vi "sub_test_lut.vi"(9 "Calibration data":T1, 10 "Normalized axis positions":sgl[](array[numeric]) format="%#.4f", 11 "Error stop":sgl=50.0) -> (2 "Plausible point":bool, 3 "Error squared":sgl[](array[numeric]) format="%#.0f")   [LabVIEW 2012]
uses:
  initialization/asap_calibration.ctl
  <vilib>/Analysis/Matrix/Datatypes/RealMatrix.ctl
  <vilib>/Analysis/Matrix/NI_Matrix.lvlib
panel:
  out "Output f(x)":sgl[](array[numeric]) format="%#.0f"
  out "XYZ and match error":sgl[](array[numeric]) format="%#.0f"
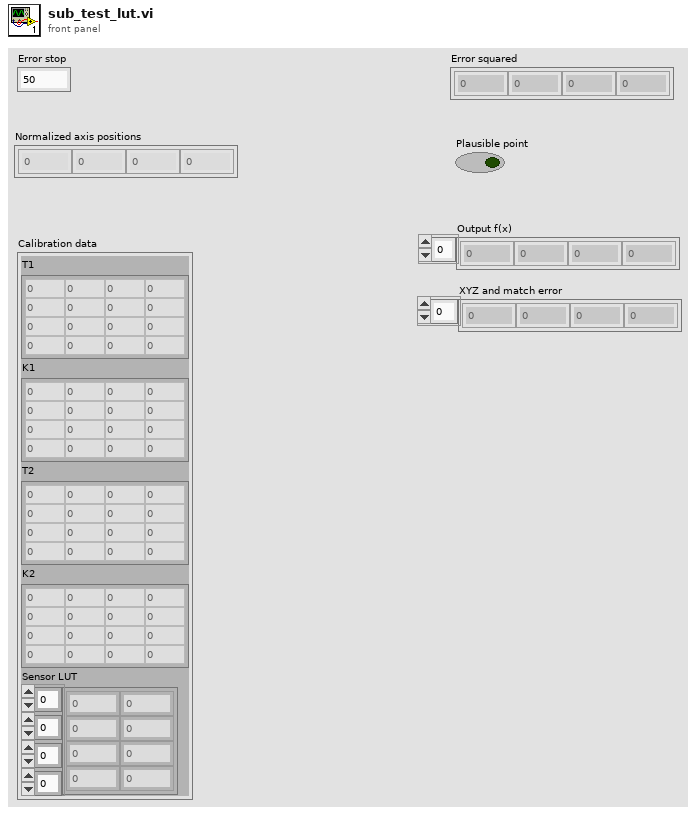
[diagram p1: front panel]
types:
  T1 = typedef "asap_calibration.ctl" = cluster{"T1":T2, "K1":T2, "T2":T2, "K2":T2, "Sensor LUT":sgl[][][][]}
  T2 = typedef "NI_Matrix.lvlib/RealMatrix.ctl" = dbl[][]
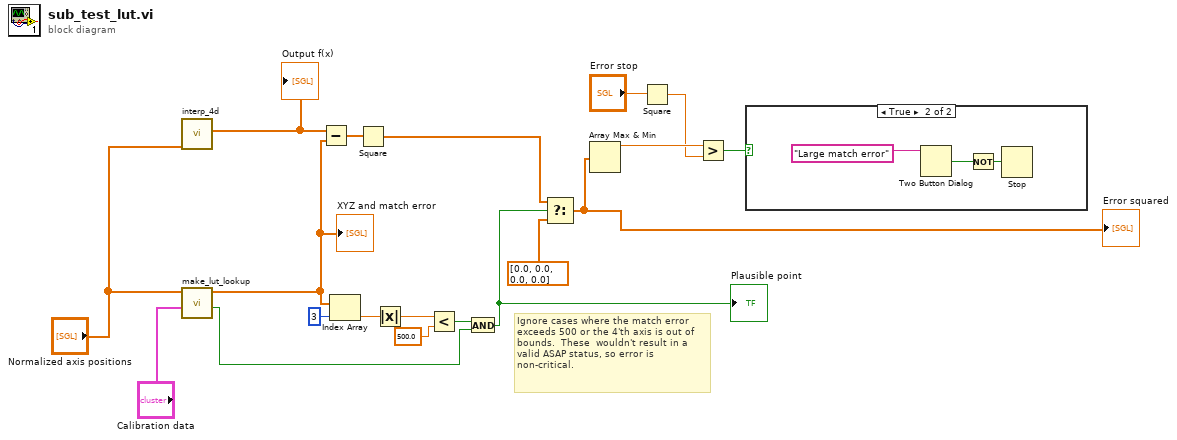
[diagram p0: block diagram]
diagram:
  # "Ignore cases where the match error exceeds 500 or the 4'th axis is out of bounds.  These  wouldn't result in a valid ASAP status, so error is non-critical."
  n1 = call "interp_4d.vi"("Input x"="Normalized axis positions") -> ("Output f(x)"=w9:sgl[])  [unwired: 10 in]
  "Output f(x)" <- w9
  n2 = call "make_lut_lookup.vi"("Calibration data"="Calibration data", "LUT inputs"="Normalized axis positions") -> ("In range"=w13:bool, "XYZ and match error"=w6:sgl[])  [unwired: 8 in]
  "XYZ and match error" <- w6
  n3 = Subtract(x=w9, y=w6) -> (x-y=w4:sgl[])
  n4 = Index Array(array=w6, index=3) -> (element=w18:sgl)
  n5 = Square(x=w4) -> (x^2=w5:sgl[])
  n6 = Absolute Value(x=w18) -> (abs(x)=w17:sgl)
  n7 = Less?(x=w17, y=sgl 500.0) -> (x < y?=w7:bool)
  n8 = And(x=w7, y=w13) -> (x .and. y?=w14:bool)
  "Plausible point" <- w14
  n9 = Select(t=w5, s=w14, f=sgl[] [0.0, 0.0, 0.0, 0.0] ("Array 2")) -> (s? t:f=w19:sgl[])
  "Error squared" <- w19
  n10 = Array Max & Min(array=w19) -> (max value=w10:sgl)  [unwired: 3 out]
  n11 = Square(x="Error stop") -> (x^2=w1:sgl)
  n12 = Greater?(x=w10, y=w1) -> (0:w11:bool)
  n13 = case shown="True" w11 {
    frame False {
    }
    frame True {
      n14 = Two Button Dialog(message="Large match error") -> (T button?=w21:bool)  [unwired: 2 in]
      n15 = Not(x=w21) -> (.not. x?=w20:bool)
      n16 = Stop(stop? (T)=w20) -> ()
    }
  }
